vi "Arithmetics_result.vi"(11 "Operation.lvclass":refnum<class "Operation.lvclass">) -> (3 "Result.lvclass 2":refnum<class "Result.lvclass">)   [LabVIEW 2024]
uses:
  Operation.lvclass
  Result/Result.lvclass
panel:
  out "Result":dbl
  in  "Result.lvclass":refnum<class "Result.lvclass">
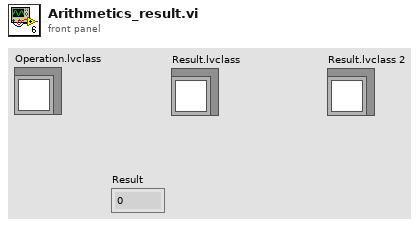
[diagram p1: front panel]
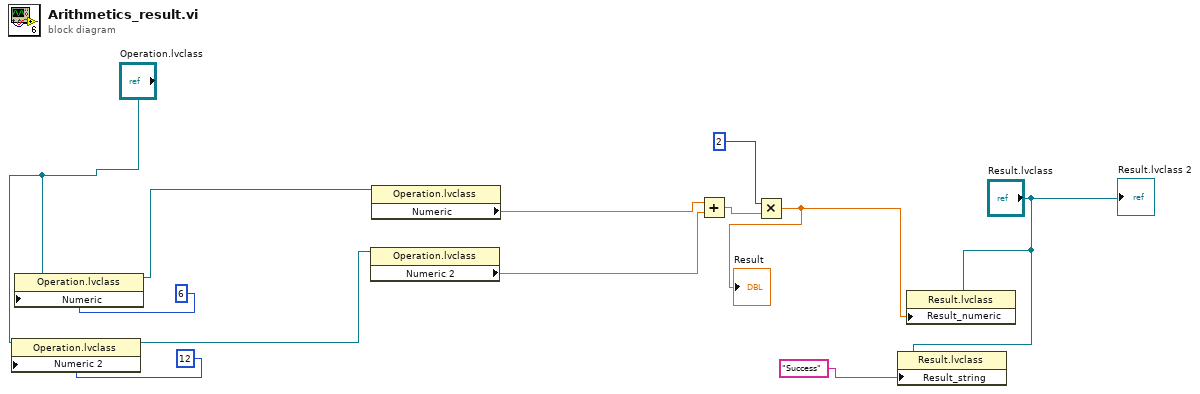
[diagram p0: block diagram]
diagram:
  n1 = property class="Operation.lvclass"(reference="Operation.lvclass", "Numeric 2"=12) -> (reference out=w3:refnum<class "Operation.lvclass">)  [unwired: 1 in, 1 out]
  n2 = property class="Operation.lvclass"(reference="Operation.lvclass", "Numeric"=6) -> (reference out=w4:refnum<class "Operation.lvclass">)  [unwired: 1 in, 1 out]
  n3 = property class="Operation.lvclass"(reference=w3) -> ("Numeric 2"=w10:dbl)  [unwired: 1 in, 2 out]
  n4 = property class="Operation.lvclass"(reference=w4) -> ("Numeric"=w11:dbl)  [unwired: 1 in, 2 out]
  n5 = Add(x=w11, y=w10) -> (x+y=w8:dbl)
  n6 = Multiply(x=2, y=w8) -> (x*y=w2:dbl)
  "Result" <- w2
  n7 = property class="Result.lvclass"(reference="Result.lvclass", "Result_string"="Success") -> ()  [unwired: 1 in, 2 out]
  n8 = property class="Result.lvclass"(reference="Result.lvclass", "Result_numeric"=w2) -> ()  [unwired: 1 in, 2 out]
  "Result.lvclass 2" <- "Result.lvclass"
